vi "generate default path.vi"(11 "current file path":path) -> (3 "browse path":path)   [LabVIEW 2013, in "Advanced Configuration Tool.lvlib"]
doc: "Generates a default file path, if the current path is empty or invalid"
uses:
  Advanced Configuration Tool.lvlib
  <vilib>/Utility/sysdir.llb/System Directory Type.ctl
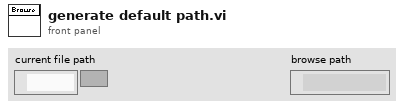
[diagram p1: front panel]
types:
  T1 = typedef "System Directory Type.ctl" = i32
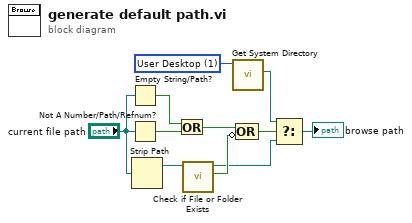
[diagram p0: block diagram]
diagram:
  w11 = T1 1 items=["User Home"=0, "User Desktop"=1, "User Documents"=2, "User Application Data"=3, "User Preferences"=4, "User Temporary"=5, "Public Documents"=6, "Public Application Data"=7, "Public Preferences"=8, "Public Cache"=13, "System Core Libraries"=9, "System Installed Libraries"=10, "Application Files"=11, "Boot Volume Root"=12] ("system directory type")
  n1 = Empty String/Path?(string/path="current file path") -> (empty?=w9:bool)
  n2 = Not A Number/Path/Refnum?(number/path/refnum="current file path") -> (NaN/Path/Refnum?=w10:bool)
  n3 = Strip Path(path="current file path") -> (stripped path=w6:path)  [unwired: 1 out]
  n4 = Or(x=w9, y=w10) -> (x .or. y?=w5:bool)
  n5 = call <vilib>:"Check if File or Folder Exists.vi"("path"=w6) -> ("file or folder exists?"=w4:bool, "dup path"=w2:path)  [unwired: 8 in, 1 out]
  n6 = call <vilib>:"Get System Directory.vi"("system directory type"=w11) -> ("system directory"=w8:path)  [unwired: 10 in]
  n7 = Compound Arithmetic op=OR(w5, invert w4) -> (w3:bool)
  n8 = Select(t=w8, s=w3, f=w2) -> (s? t:f=→"browse path":path)
